vi "Execute Open DQMH Request Message Diagram QD.vi"(6 "Mouse Position":T1, 8 "User VI Ref":refnum<vi>, 9 "Menu Item Tag Suffix":string, 10 "Remaining Items":refnum<vi>[](array[refnum]), 11 "Affected Items":T2) -> (0 "Fail transaction?":bool)   [LabVIEW 2017]
doc: "This VI is part of a plug-in for modifying the LabVIEW shortcut menus. This is the execute VI which is called when the shortcut menu is chosen by the user. It performs the action of the selected menu item."
uses:
  plugins/PopupMenus/edit time panel and diagram/Open DQMH Request Message Diagram.llb/Open DQMH Request Message Diagram.ctl
  <vilib>/Utility/miscctls.llb/LVPositionTypeDef.ctl
panel:
  # "All controls on this panel except \"Affected Items\" have been locked to prevent accidental edits. Changing the control names or types, other than the elements of the \"Affected Items\" cluster will make the VI unusable as a menu plugin.\n\nSee Context Help for each control for details about its use."
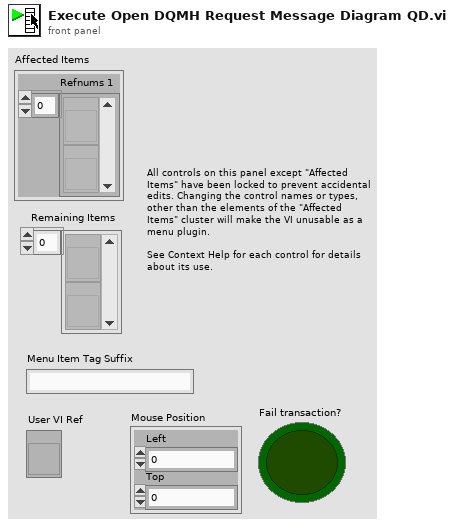
[diagram p1: front panel]
types:
  T1 = typedef "LVPositionTypeDef.ctl" = cluster{"Left":i32, "Top":i32}
  T2 = typedef "Open DQMH Request Message Diagram.ctl" = cluster{"Refnums 1":refnum<vi>[]}
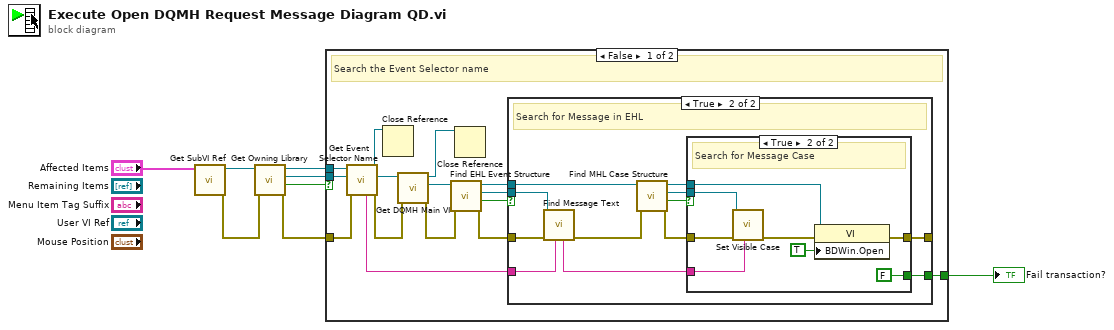
[diagram p0: block diagram]
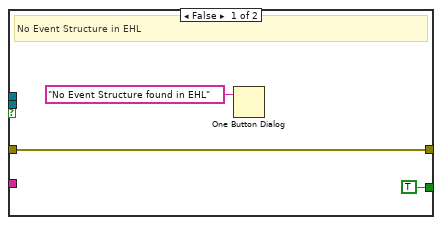
[diagram p2: hidden frame]
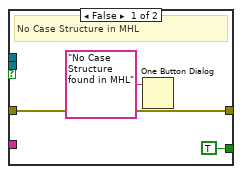
[diagram p3: hidden frame]
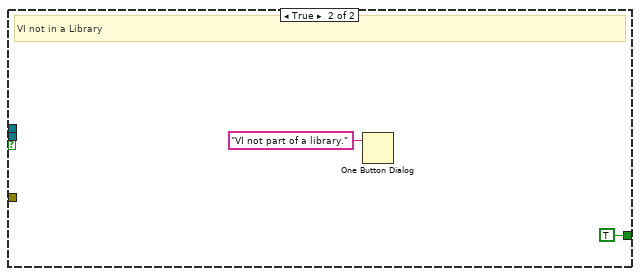
[diagram p4: hidden frame]
diagram:
  n1 = call "Get SubVI Ref.vi"("Affected Items"="Affected Items") -> ("error out"=w6:errorcluster, "Selected SubVI Reference"=w7:refnum<vi>)  [unwired: 9 in]
  n2 = call "Get Owning Library.vi"("error in (no error)"=w6, "VI in"=w7) -> ("error out"=w4:errorcluster, "Not In Library"=w1:bool, "Owning Library"=w3:refnum<vi>, "VI out"=w5:refnum<vi>)  [unwired: 6 in]
  n3 = case shown="False" w1 {
    tunnel: w5 -> [w23 _]
    tunnel: w4 -> [w22 _]
    tunnel: w3 -> [w21 _]
    tunnel: [w12 TRUE ("Fail transaction?")] -> w2
    frame False {
      # "Search the Event Selector name"
      n4 = call "Get Event Selector Name.vi"("error in (no error)"=w22, "Library Ref in"=w21, "VI Ref in"=w23) -> ("error out"=w19:errorcluster, "Library Ref out"=w20:refnum<vi>, "VI Ref out"=w9:refnum<vi>, "Event Selector Name"=w13:string)  [unwired: 5 in]
      n5 = Close Reference(reference=w9) -> ()  [unwired: 1 in, 1 out]
      n6 = call "Get DQMH Main VI.vi"("error in (no error)"=w19, "Library Ref in"=w20) -> ("error out"=w17:errorcluster, "Main VI Ref"=w11:refnum<vi>, "Library Ref out"=w10:refnum<vi>)  [unwired: 7 in]
      n7 = call "Find EHL Event Structure.vi"("error in (no error)"=w17, "VI Ref in"=w11) -> ("error out"=w18:errorcluster, "Found?"=w14:bool, "EHL Event Structure"=w16:refnum<vi>, "VI Ref out"=w15:refnum<vi>)  [unwired: 6 in]
      n8 = Close Reference(reference=w10) -> ()  [unwired: 1 in, 1 out]
      n9 = case shown="True" w14 {
        tunnel: w13 -> [_ w38]
        tunnel: w18 -> [w26 w37]
        tunnel: w16 -> [_ w36]
        tunnel: w15 -> [_ w35]
        tunnel: [w26 w31] -> _
        tunnel: [TRUE ("Fail transaction?") w27] -> w12
        frame False {
          # "No Event Structure in EHL"
          n10 = One Button Dialog(message="No Event Structure found in EHL") -> ()  [unwired: 1 in, 1 out]
        }
        frame True {
          # "Search for Message in EHL"
          n11 = call "Find Message Text.vi"("Event Selector Name"=w38, "error in (no error)"=w37, "EventStructure in"=w36) -> ("error out"=w34:errorcluster, "Message Text"=w30:string)  [unwired: 7 in]
          n12 = call "Find MHL Case Structure.vi"("error in (no error)"=w34, "VI Ref in"=w35) -> ("error out"=w32:errorcluster, "Found?"=w29:bool, "MHL Case Structure"=w33:refnum<vi>, "VI Ref out"=w28:refnum<vi>)  [unwired: 6 in]
          n13 = case shown="True" w29 {
            tunnel: w33 -> [_ w49]
            tunnel: w32 -> [w41 w48]
            tunnel: [w41 w43] -> w31
            tunnel: w30 -> [_ w47]
            tunnel: w28 -> [_ w45]
            tunnel: [TRUE ("Fail transaction?") FALSE ("Fail transaction?")] -> w27
            frame False {
              # "No Case Structure in MHL"
              n14 = One Button Dialog(message="No Case Structure found in MHL") -> ()  [unwired: 1 in, 1 out]
            }
            frame True {
              # "Search for Message Case"
              n15 = call "Set Visible Case.vi"("Message Text"=w47, "error in (no error)"=w48, "CaseStructure in"=w49) -> ("error out"=w44:errorcluster)  [unwired: 8 in]
              n16 = property class="VI"(reference=w45, error in=w44, "BDWin.Open"=TRUE ("Block Diagram Window:Open")) -> (error out=w43:errorcluster)  [unwired: 1 out]
            }
          }
        }
      }
    }
    frame True {
      # "VI not in a Library"
      n17 = One Button Dialog(message="VI not part of a library.") -> ()  [unwired: 1 in, 1 out]
    }
  }
  "Fail transaction?" <- w2
